vi "WaveGenerator_Sample_Program.vi"(0 "System no.":i32=1 min=1 step=1, 1 "Stop refnum":refnum<vi>, 2 "Affected axis":string="1", 3 "Selection":T1, 4 "DDL":bool, 5 "error in":errorcluster, 6 "Sine Parameters:":T3={"Xo (Start)"=0, "SIN_P Parameters"={"C"=200.0, "A"=10.0, "O"=0.0}, "N (Length)"=500, "Append? (&)"=FALSE} {"N (Length)" min=0 max=1000 step=1; "SIN_P Parameters"."O" format="%.6f"; "SIN_P Parameters"."A" format="%.6f"; "SIN_P Parameters"."C" format="%.6f"}, 7 "Ramp Parameters:":T2={"Xo (Start)"=0, "RAMP Parameters"={"C"=200.0, "J"=0.0, "A"=8.0, "O"=0.0}, "N (Length)"=500, "Append? (&)"=FALSE} {"N (Length)" min=0 max=1000 step=1; "RAMP Parameters"."O" format="%.6f"; "RAMP Parameters"."A" format="%.6f"; "RAMP Parameters"."J" format="%.6f"; "RAMP Parameters"."C" format="%.6f"}, 8 "Start position":dbl format="%.6f") -> (14 "Waveform":dbl[][](graph) caption="Graph showing the commanded (green) and measured (white) waveform and the position error (red).", 19 "Error out":errorcluster)   [LabVIEW 2014]
doc: "This VI demonstrates how to use the wave generator command VIs. It first moves the affected axis to a given start position. Then it runs in a loop, giving the user the options to write sine wave curve segments or ramps into the controllers wave buffer. Wave storage data points are limited to 1000 points to keep transfer times low. The segment length of one waveform - which normally defines the frequency - is predefined as 500 points in this example. Depending on the value of Append? (&), either the old buffer data is overwritten or the new wave will be appended to memory. Please take into account that you can append at most two waveforms since buffer size is limited to 1000 points as mentioned above. \n\nAdjust the following controls to modify the shape of the waveforms.\nN (Length): Waveform (i.e. the points to be modified) goes from 1 to Length. Datapoints from Length to 500 are filled with value of last wave point.\nXo (Start): Position where the first point of the waveform is located. \nC: Center point of the wave. If C = Length/2 then the wave is symmetrical.\nA: Amplitude of the waveform. F(x) = A*sin(x) + O\nO: Offset of the waveform. F(x) = A*sin(x) + O\nJ: Jerk. Means curvature in the transition to or from standstill.\n\nYou have to stop generator output prior to restarting it with a different parameter set. The Start Gen. and Stop Gen. buttons will enable or disable the wave generator output by sending \"WGO 0\" or \"WGO 1\" for the affected axis. If DDL is enabled \"WGO 65\" will be sent respectively. The red Stop button stops the wave generator output on the specified axis and finishes the loop. Please respect the delays that occur while the controller is processing your commands. This is indicated by the \"Busy?\" indicator. See manual for further details. \n\nIn case of an error a button Clear Error will appear and the control buttons above will be disabled. Pressing this button will clear the error status and enable the control buttons again.\nWith DDL ON you can achieve significantly better position accuracy. Compare the target (green), response (white) and error (red) signals on the graph. Since this is a very sensitive mechanism we recommend starting with low amplitudes and adjusting the parameters with caution. The DDL button works only if the controller supports DDL. Contact PI for information on activation of DDL support.\n\nSee User Manual for details about the use of the wave generator.\n\nRun XXXX_Configuration_Setup (with XXXX being the product number of your PI controller) prior to running this VI.\n\nValid for: E-712, E-725, E-727, E-753, E-754"
panel:
  out "Gen. running?":bool
  out "DDL":bool
  in  "Clear Error":bool
  out "Busy?":bool
  out "Controller error":bool
  in  "Stop":bool
  # "Wave generator sample program"
  # "This VI demonstrates how to use the wave generator command VIs. It first moves the affected axis to a given start position. Then it runs in a loop, giving the\nuser the options to write sine wave curve segments or ramps into the controllers wave buffer. Wave storage data points are limited to 1000 points\nto keep transfer times low. The segment length of one waveform is predefined as 500 points in this example. Depending on the value of Append? (&), either\nthe old buffer data is overwritten or the new wave will be appended to memory. You have to stop generator output prior to restarting it with a different\nparameter set. The Start Gen. and Stop Gen. buttons will enable or disable the wave generator output by sending \"WGO 0\" or \"WGO 1\" for the affected axis. \nIf DDL is enabled \"WGO 65\" will be sent respectively. The red Stop button stops the wave generator output on the specified axis and finishes the loop. Please\nrespect the delays that occur while the controller is processing your commands. This is indicated by the \"Busy?\" indicator. See manual for further details. \nRun XXXX_Configuration_Setup (with XXXX being the product number of your PI controller) prior to running this VI."
  # "DDL state"
  # "Stop VI\nand wave\ngenerator\noutput"
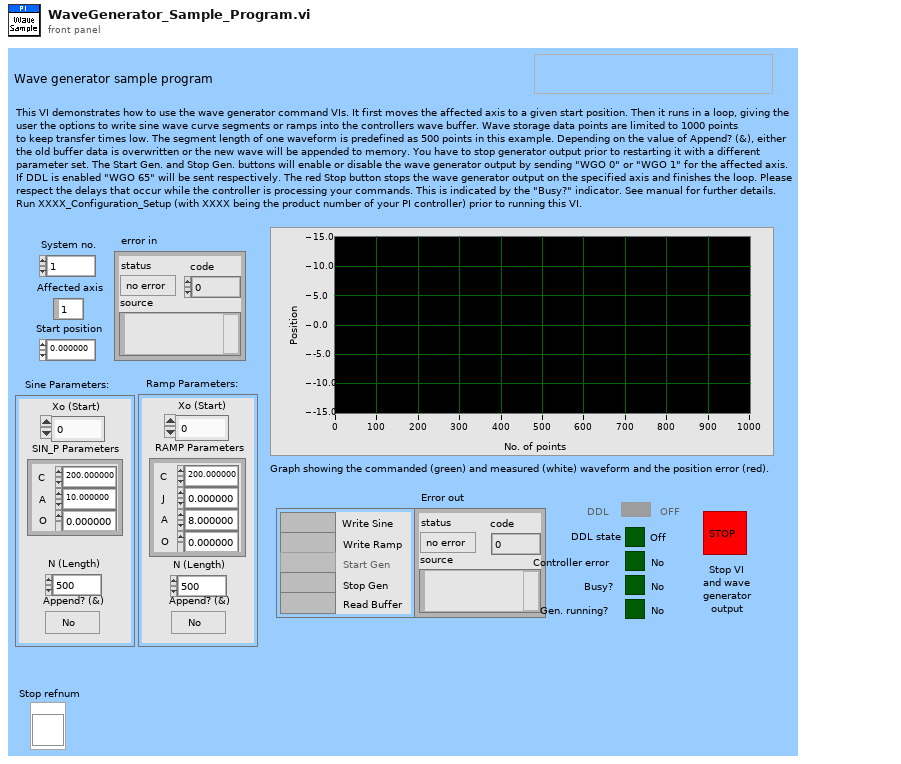
[diagram p1: front panel]
types:
  T1 = cluster{"Write Sine":bool, "Write Ramp":bool, "Start Gen":bool, "Stop Gen":bool, "Read Buffer":bool}
  T2 = cluster{"Xo (Start)":i32, "RAMP Parameters":cluster{"C":dbl, "J":dbl, "A":dbl, "O":dbl}, "N (Length)":i32, "Append? (&)":bool}
  T3 = cluster{"Xo (Start)":i32, "SIN_P Parameters":cluster{"C":dbl, "A":dbl, "O":dbl}, "N (Length)":i32, "Append? (&)":bool}
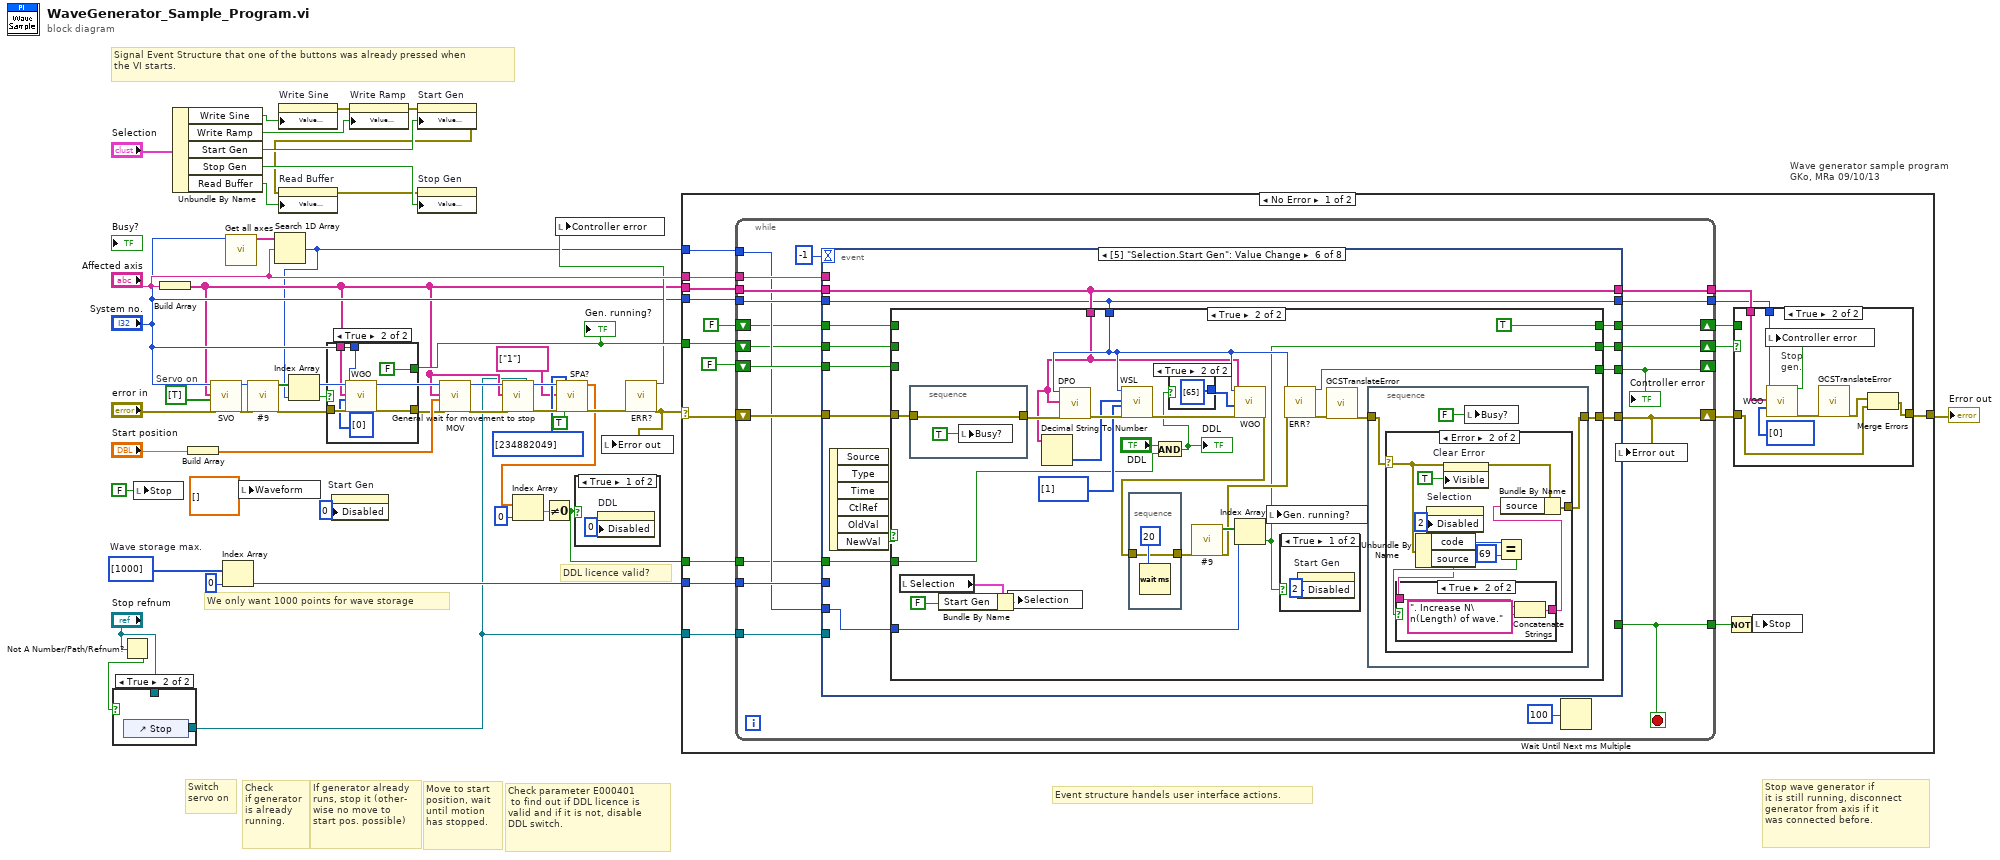
[diagram p0: block diagram]
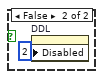
[diagram p2: hidden frame]
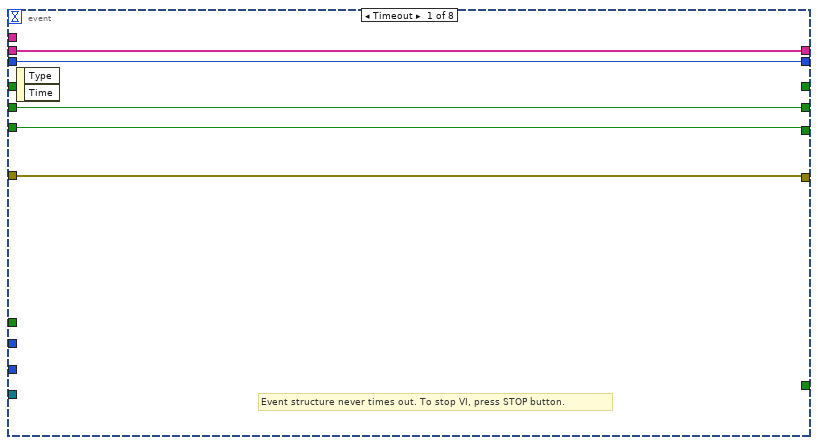
[diagram p6: hidden frame]
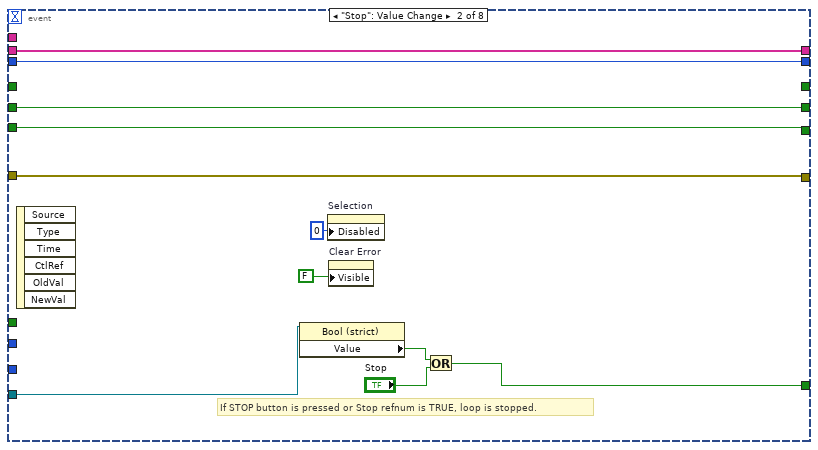
[diagram p7: hidden frame]
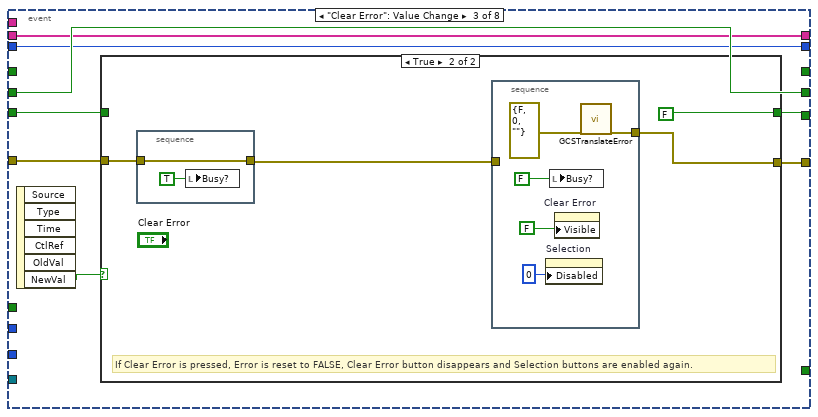
[diagram p8: hidden frame]
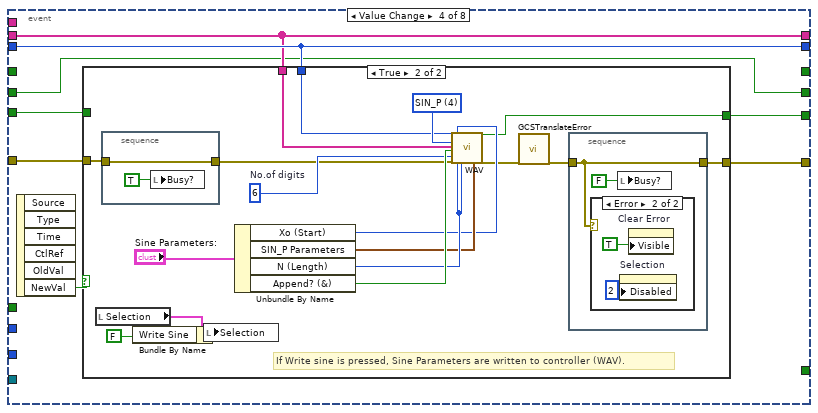
[diagram p10: hidden frame]
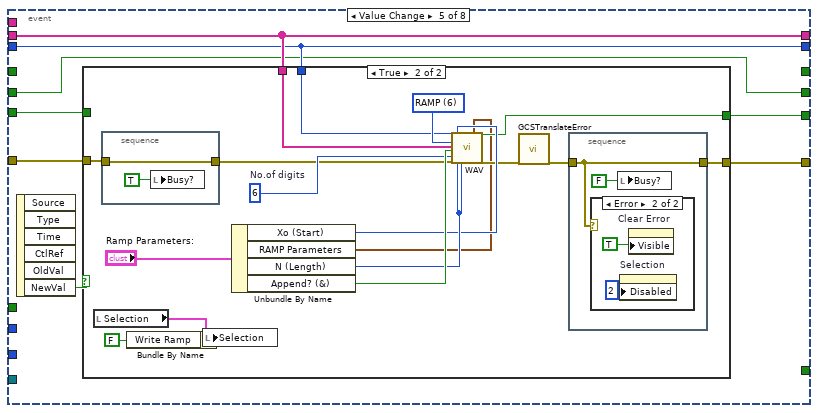
[diagram p13: hidden frame]
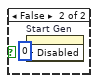
[diagram p17: hidden frame]
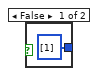
[diagram p18: hidden frame]
diagram:
  w44 = i32[] [1000]  # Wave storage max.
  # "Stop wave generator if\nit is still running, disconnect \ngenerator from axis if it\nwas connected before."
  # "Event structure handels user interface actions."
  # "Check parameter E000401\n to find out if DDL licence is\nvalid and if it is not, disable\nDDL switch."
  # "If generator already\nruns, stop it (other-\nwise no move to\nstart pos. possible)"
  # "Check\nif generator\nis already \nrunning."
  # "We only want 1000 points for wave storage"
  # "Switch\nservo on"
  # "Signal Event Structure that one of the buttons was already pressed when\nthe VI starts."
  # "DDL licence valid?"
  # "Servo on"
  # "Move to start\nposition, wait\nuntil motion\nhas stopped."
  # "Wave generator sample program\nGKo, MRa 09/10/13"
  n1 = Not A Number/Path/Refnum?(number/path/refnum="Stop refnum") -> (NaN/Path/Refnum?=w40:bool)
  n2 = case shown="True" w40 {
    tunnel: [w48 w49] -> w6
    tunnel: "Stop refnum" -> [w48 _]
    frame False {
    }
    frame True {
      n3 = control-ref of="Stop"() -> (w49:refnum<vi>)
    }
  }
  n4 = local write "Stop"(FALSE ("Controller error")) -> ()
  n5 = Build Array("Affected axis") -> (w20:string[])
  n6 = Unbundle By Name("Selection") -> ("Write Sine"=w11:bool, "Write Ramp"=w10:bool, "Start Gen"=w9:bool, "Stop Gen"=w8:bool, "Read Buffer"=w7:bool)
  n7 = Build Array("Start position") -> (w41:dbl[])
  n8 = call "SVO.vi"("System no."="System no.", "Axes to command"=w20, "Servo mode"=bool[] [TRUE], "error in"="error in") -> ("error out"=w34:errorcluster)  [unwired: 1 in, 14 out]
  n9 = Index Array(array=w44, index=0 ("Index")) -> (element=w45:i32)
  n10 = call "Get all axes.vi"("System no."="System no.") -> ("Conn. Axes"=w36:string[])  [unwired: 18 out]
  n11 = local write "Waveform"(dbl[][] [] ("Waveform")) -> ()
  n12 = call "#9.vi"("System no."="System no.", "error in"=w34) -> ("WG running?"=w37:bool[], "error out"=w29:errorcluster)  [unwired: 16 out]
  n13 = Search 1D Array(1D array=w36, element="Affected axis") -> (index of element=w16:i32)  [unwired: 1 out]
  n14 = property on="Write Sine" class="Bool (strict)"("Value (Signaling)"=w11) -> (error out=w5:errorcluster)  [unwired: 2 in, 1 out]
  n15 = Index Array(array=w37, index=w16) -> (element=w30:bool)
  n16 = case shown="True" w30 {
    selector: w30 -> [w51 _]
    tunnel: w29 -> [w50 w57]
    tunnel: [w50 w56] -> w28
    tunnel: "System no." -> [_ w54]
    tunnel: w20 -> [_ w53]
    tunnel: [w51 FALSE] -> w27
    frame False {
    }
    frame True {
      n17 = call "WGO.vi"("System no."=w54, "Affected axes"=w53, "WGO Parameter"=i32[] [0], "error in"=w57) -> ("error out"=w56:errorcluster)  [unwired: 15 out]
    }
  }
  "Gen. running?" <- w27
  n18 = property on="Start Gen" class="Bool (strict)"("Disabled"=u8 0) -> ()  [unwired: 2 in, 2 out]
  n19 = property on="Write Ramp" class="Bool (strict)"(error in=w5, "Value (Signaling)"=w10) -> (error out=w4:errorcluster)  [unwired: 1 in, 1 out]
  n20 = property on="Start Gen" class="Bool (strict)"(error in=w4, "Value (Signaling)"=w9) -> (error out=w3:errorcluster)  [unwired: 1 in, 1 out]
  n21 = property on="Stop Gen" class="Bool (strict)"(error in=w3, "Value (Signaling)"=w8) -> (error out=w2:errorcluster)  [unwired: 1 in, 1 out]
  n22 = property on="Read Buffer" class="Bool (strict)"(error in=w2, "Value (Signaling)"=w7) -> ()  [unwired: 1 in, 2 out]
  n23 = call "MOV.vi"("System no."="System no.", "Axes to move"=w20, "Position values"=w41, "error in"=w28) -> ("error out"=w31:errorcluster)  [unwired: 1 in, 14 out]
  n24 = call "General wait for movement to stop.vi"("System no."="System no.", "Axes to wait for"=w20, "error in"=w31, "Stop refnum"=w6) -> ("error out"=w22:errorcluster)  [unwired: 4 in, 11 out]
  n25 = call "SPA?.vi"("System no."="System no.", "Axes to query"=string[] ["1"], "error in"=w22, "Parameter no. (hex)"=u32[] [234882049], "Parameter no. format \n(Decimal: FALSE)"=TRUE ("Parameter no. format \n(Decimal: FALSE)")) -> ("Parameter value"=w17:dbl[], "error out"=w23:errorcluster)  [unwired: 2 in, 11 out]
  n26 = Index Array(array=w17, index=0) -> (element=w14:dbl)
  n27 = Not Equal To 0?(x=w14) -> (x != 0?=w13:bool)
  n28 = case shown="True" w13 {
    frame True {
      n29 = property on="DDL" class="Bool (strict)"("Disabled"=u8 0) -> ()  [unwired: 2 in, 2 out]
    }
    frame False {
      n30 = property on="DDL" class="Bool (strict)"("Disabled"=u8 2) -> ()  [unwired: 2 in, 2 out]
    }
  }
  n31 = call "ERR?.vi"("error in"=w23) -> ("Controller error"=w25:bool, "error out"=w26:errorcluster)  [unwired: 1 in, 16 out]
  n32 = local write "Controller error"(w25) -> ()
  n33 = local write "Error out"(w26) -> ()
  n34 = case shown="No Error" w26 {
    selector: w26 -> [w70 w376]
    tunnel: w20 -> [w78 _]
    tunnel: "System no." -> [w77 _]
    tunnel: [w68 w375] -> w47
    tunnel: w45 -> [w71 _]
    tunnel: "Affected axis" -> [w73 _]
    tunnel: w16 -> [w69 _]
    tunnel: w27 -> [w67 _]
    tunnel: w13 -> [w61 _]
    tunnel: w6 -> [w60 _]
    frame No Error {
      n35 = while {
        tunnel: w73 -> [w99]
        tunnel: w71 -> [w100]
        shift-left: w70 -> [w102]
        shift-right: [w101] -> w74
        tunnel: [w103] -> w75
        tunnel: [w105] -> w76
        tunnel: w77 -> [w104]
        tunnel: w78 -> [w106]
        shift-right: [w97] -> _
        shift-left: FALSE ("Controller error") -> [w96]
        tunnel: w69 -> [w95]
        shift-right: [w93] -> w66
        shift-left: w67 -> [w94]
        tunnel: [w92] -> w65
        shift-right: [w91] -> w62
        shift-left: FALSE -> [w90]
        tunnel: w61 -> [w89]
        tunnel: w60 -> [w88]
        stop <- w92 stop-if-true
        n36 = event shown="[5] \"Selection.Start Gen\": Value Change" {
          selector: _ -> [_ _ _ _ _ _ _ _]
          dyn-events: _ -> [_ _ _ _ _ _ _ _]
          timeout: -1 -> [_ _ _ _ _ _ _ _]
          tunnel: w106 -> [w110 w121 w124 w146 w181 w220 w284 w323]
          tunnel: [w110 w121 w124 w146 w181 w220 w284 w323] -> w105
          tunnel: w104 -> [w109 w120 w125 w147 w180 w219 w283 w324]
          tunnel: [w109 w120 w125 w147 w180 w219 w283 w324] -> w103
          tunnel: w102 -> [w111 w122 w127 w150 w184 w223 w288 w330]
          tunnel: [w111 w122 w128 w151 w185 w224 w289 w331] -> w101
          tunnel: w100 -> [_ _ _ _ _ _ _ w325]
          tunnel: w99 -> [_ _ _ _ _ _ _ w326]
          tunnel: [w112 w123 w129 w152 w186 w225 w290 w332] -> w97
          tunnel: w96 -> [w112 w123 w130 w148 w182 w221 w286 w328]
          tunnel: w95 -> [_ _ _ _ _ w213 w285 w327]
          tunnel: [_ w115 _ _ _ _ _ _] -> w92
          tunnel: w94 -> [w108 w119 w126 w145 w179 w217 w281 w322]
          tunnel: [w108 w119 w126 w145 w179 w218 w282 w322] -> w93
          tunnel: [_ _ _ _ _ w216 _ _] -> w91
          tunnel: w90 -> [_ _ _ _ _ w215 _ _]
          tunnel: w89 -> [_ _ _ _ _ w214 _ _]
          tunnel: w88 -> [_ w118 _ _ _ _ _ _]
          event Timeout {
            # "Event structure never times out. To stop VI, press STOP button."
            n37 = event-data() -> ()  [unwired: 3 out]
          }
          event "Stop": Value Change {
            # "If STOP button is pressed or Stop refnum is TRUE, loop is stopped."
            n38 = event-data() -> ()  [unwired: 7 out]
            n39 = property class="Bool (strict)"(reference=w118) -> ("Value"=w117:bool)  [unwired: 1 in, 2 out]
            n40 = property on="Selection" class="Clust (strict)"("Disabled"=u8 0) -> ()  [unwired: 2 in, 2 out]
            n41 = property on="Clear Error" class="Bool"("Visible"=FALSE) -> ()  [unwired: 2 in, 2 out]
            n42 = Or(x=w117, y="Stop") -> (x .or. y?=w115:bool)
          }
          event "Clear Error": Value Change {
            n43 = event-data() -> ("NewVal"=w131:bool)  [unwired: 6 out]
            n44 = case shown="True" w131 {
              tunnel: w130 -> [w133 _]
              tunnel: [w133 FALSE ("Controller error")] -> w129
              tunnel: [w132 w135] -> w128
              tunnel: w127 -> [w132 w136]
              frame False {
              }
              frame True {
                # "If Clear Error is pressed, Error is reset to FALSE, Clear Error button disappears and Selection buttons are enabled again."
                n45 = stacked-sequence {
                  tunnel: w136 -> [w143]
                  tunnel: [w143] -> w134
                  frame #0 {
                    n46 = local write "Busy?"(TRUE) -> ()
                  }
                }
                n47 = stacked-sequence {
                  tunnel: [w138] -> w135
                  tunnel: w134 -> [_]
                  frame #0 {
                    n48 = property on="Selection" class="Clust (strict)"("Disabled"=u8 0) -> ()  [unwired: 2 in, 2 out]
                    n49 = local write "Busy?"(FALSE) -> ()
                    n50 = property on="Clear Error" class="Bool"("Visible"=FALSE) -> ()  [unwired: 2 in, 2 out]
                    n51 = call "GCSTranslateError.vi"("error in"=errorcluster {"status"=FALSE, "code"=0, "source"=""} ("error IO")) -> ("error out"=w138:errorcluster)  [unwired: 18 out]
                  }
                }
              }
            }
          }
          event "Selection.Write Sine": Value Change {
            n52 = event-data() -> ("NewVal"=w149:bool)  [unwired: 6 out]
            n53 = case shown="True" w149 {
              tunnel: [w153 w165] -> w152
              tunnel: w147 -> [_ w157]
              tunnel: w146 -> [_ w156]
              tunnel: [w154 w162] -> w151
              tunnel: w150 -> [w154 w161]
              tunnel: w148 -> [w153 _]
              frame False {
              }
              frame True {
                w168 = i16 6  # No.of digits
                w167 = u16 4 items=["SIN", "POL", "TAN", "PNT", "SIN_P", "LIN", "RAMP"] ("Waveform")
                # "If Write sine is pressed, Sine Parameters are written to controller (WAV)."
                n54 = local read "Selection"() -> (w160:T1)
                n55 = stacked-sequence {
                  tunnel: w161 -> [w173]
                  tunnel: [w173] -> w155
                  frame #0 {
                    n56 = local write "Busy?"(TRUE) -> ()
                  }
                }
                n57 = Bundle By Name(cluster=w160, "Write Sine"=FALSE) -> (w159:T1)
                n58 = local write "Selection"(w159) -> ()
                n59 = Unbundle By Name("Sine Parameters:") -> ("Xo (Start)"=w169:i32, "SIN_P Parameters"=w170:cluster{"C":dbl, "A":dbl, "O":dbl}, "N (Length)"=w171:i32, "Append? (&)"=w172:bool)
                n60 = call "WAV.vi"("System no."=w157, "Waveform"=w167, "Affected axes"=w156, "Append? (&)"=w172, "No.of digits"=w168, "error in"=w155, "Xo"=w169, "N"=w171, "Segment length"=w171, "SIN_P Parameters"=w170) -> ("Controller error"=w165:bool, "error out"=w164:errorcluster)  [unwired: 10 in, 6 out]
                n61 = call "GCSTranslateError.vi"("error in"=w164) -> ("error out"=w163:errorcluster)  [unwired: 18 out]
                n62 = stacked-sequence {
                  tunnel: w163 -> [w175]
                  tunnel: [w175] -> w162
                  frame #0 {
                    n63 = case shown="Error" w175 {
                      frame No Error {
                      }
                      frame Error {
                        n64 = property on="Selection" class="Clust (strict)"("Disabled"=u8 2) -> ()  [unwired: 2 in, 2 out]
                        n65 = property on="Clear Error" class="Bool"("Visible"=TRUE) -> ()  [unwired: 2 in, 2 out]
                      }
                    }
                    n66 = local write "Busy?"(FALSE) -> ()
                  }
                }
              }
            }
          }
          event "Selection.Write Ramp": Value Change {
            n67 = event-data() -> ("NewVal"=w183:bool)  [unwired: 6 out]
            n68 = case shown="True" w183 {
              tunnel: [w187 w201] -> w186
              tunnel: w180 -> [_ w200]
              tunnel: w181 -> [_ w199]
              tunnel: [w188 w196] -> w185
              tunnel: w184 -> [w188 w195]
              tunnel: w182 -> [w187 _]
              frame False {
              }
              frame True {
                w203 = i16 6  # No.of digits
                w202 = u16 6 items=["SIN", "POL", "TAN", "PNT", "SIN_P", "LIN", "RAMP"] ("Waveform")
                n69 = local read "Selection"() -> (w191:T1)
                n70 = stacked-sequence {
                  tunnel: w195 -> [w207]
                  tunnel: [w207] -> w194
                  frame #0 {
                    n71 = local write "Busy?"(TRUE) -> ()
                  }
                }
                n72 = Bundle By Name(cluster=w191, "Write Ramp"=FALSE ("Write Sine")) -> (w190:T1)
                n73 = local write "Selection"(w190) -> ()
                n74 = Unbundle By Name("Ramp Parameters:") -> ("Xo (Start)"=w204:i32, "RAMP Parameters"=w192:cluster{"C":dbl, "J":dbl, "A":dbl, "O":dbl}, "N (Length)"=w205:i32, "Append? (&)"=w206:bool)
                n75 = call "WAV.vi"("System no."=w200, "Waveform"=w202, "Affected axes"=w199, "Append? (&)"=w206, "No.of digits"=w203, "error in"=w194, "Xo"=w204, "N"=w205, "Segment length"=w205, "RAMP Parameters"=w192) -> ("Controller error"=w201:bool, "error out"=w198:errorcluster)  [unwired: 10 in, 6 out]
                n76 = call "GCSTranslateError.vi"("error in"=w198) -> ("error out"=w197:errorcluster)  [unwired: 18 out]
                n77 = stacked-sequence {
                  tunnel: w197 -> [w209]
                  tunnel: [w209] -> w196
                  frame #0 {
                    n78 = case shown="Error" w209 {
                      frame No Error {
                      }
                      frame Error {
                        n79 = property on="Selection" class="Clust (strict)"("Disabled"=u8 2) -> ()  [unwired: 2 in, 2 out]
                        n80 = property on="Clear Error" class="Bool"("Visible"=TRUE) -> ()  [unwired: 2 in, 2 out]
                      }
                    }
                    n81 = local write "Busy?"(FALSE) -> ()
                  }
                }
              }
            }
          }
          event "Selection.Start Gen": Value Change {
            n82 = event-data() -> ("NewVal"=w222:bool)  [unwired: 6 out]
            n83 = case shown="True" w222 {
              tunnel: [w228 w245] -> w225
              tunnel: w219 -> [_ w244]
              tunnel: w220 -> [_ w243]
              tunnel: [w229 w254] -> w224
              tunnel: w223 -> [w229 w253]
              tunnel: w221 -> [w228 _]
              tunnel: [w227 w238] -> w218
              tunnel: w217 -> [w227 _]
              tunnel: [w226 TRUE] -> w216
              tunnel: w215 -> [w226 _]
              tunnel: w214 -> [_ w232]
              tunnel: w213 -> [_ w230]
              frame False {
              }
              frame True {
                n84 = local read "Selection"() -> (w237:T1)
                n85 = stacked-sequence {
                  tunnel: w253 -> [w262]
                  tunnel: [w262] -> w247
                  frame #0 {
                    n86 = local write "Busy?"(TRUE) -> ()
                  }
                }
                n87 = Bundle By Name(cluster=w237, "Start Gen"=FALSE ("Write Sine")) -> (w236:T1)
                n88 = local write "Selection"(w236) -> ()
                n89 = Decimal String To Number(string=w243) -> (number=w248:i32[])  [unwired: 3 out]
                n90 = call "DPO.vi"("System no."=w244, "DPO axes"=w243, "error in"=w247) -> ("error out"=w250:errorcluster)  [unwired: 2 in, 14 out]
                n91 = call "WSL.vi"("System no."=w244, "Generator ID"=w248, "WaveTableID"=i32[] [1], "error in"=w250) -> ("error out"=w251:errorcluster)  [unwired: 15 out]
                n92 = And(x="DDL", y=w232) -> (x .and. y?=w231:bool)
                "DDL" <- w231
                n93 = case shown="True" w231 {
                  tunnel: [i32[] [1] ("WGO Parameter") i32[] [65] ("WGO Parameter")] -> w252
                  frame False {
                  }
                  frame True {
                  }
                }
                n94 = call "WGO.vi"("System no."=w244, "Affected axes"=w243, "WGO Parameter"=w252, "error in"=w251) -> ("error out"=w240:errorcluster)  [unwired: 15 out]
                n95 = stacked-sequence {
                  tunnel: w240 -> [w258]
                  tunnel: [w258] -> w242
                  frame #0 {
                    n96 = Wait (ms)(milliseconds to wait=u32 20) -> ()  [unwired: 1 out]
                  }
                }
                n97 = call "#9.vi"("error in"=w242) -> ("WG running?"=w241:bool[], "error out"=w239:errorcluster)  [unwired: 1 in, 16 out]
                n98 = Index Array(array=w241, index=w230) -> (element=w238:bool)
                n99 = local write "Gen. running?"(w238) -> ()
                n100 = case shown="True" w238 {
                  frame True {
                    n101 = property on="Start Gen" class="Bool (strict)"("Disabled"=u8 2) -> ()  [unwired: 2 in, 2 out]
                  }
                  frame False {
                    n102 = property on="Start Gen" class="Bool (strict)"("Disabled"=u8 0) -> ()  [unwired: 2 in, 2 out]
                  }
                }
                n103 = call "ERR?.vi"("System no."=w244, "error in"=w239) -> ("Controller error"=w245:bool, "error out"=w246:errorcluster)  [unwired: 16 out]
                n104 = call "GCSTranslateError.vi"("error in"=w246) -> ("error out"=w255:errorcluster)  [unwired: 18 out]
                n105 = stacked-sequence {
                  tunnel: w255 -> [w265]
                  tunnel: [w264] -> w254
                  frame #0 {
                    n106 = case shown="Error" w265 {
                      selector: w265 -> [w267 w272]
                      tunnel: [w267 w270] -> w264
                      frame No Error {
                      }
                      frame Error {
                        n107 = Unbundle By Name(w272) -> ("code"=w274:i32, "source"=w268:string)
                        n108 = property on="Selection" class="Clust (strict)"("Disabled"=u8 2) -> ()  [unwired: 2 in, 2 out]
                        n109 = property on="Clear Error" class="Bool"("Visible"=TRUE) -> ()  [unwired: 2 in, 2 out]
                        n110 = Equal?(x=w274, y=69) -> (x = y?=w269:bool)
                        n111 = case shown="True" w269 {
                          tunnel: [w277 w279] -> w271
                          tunnel: w268 -> [w277 w278]
                          frame False {
                          }
                          frame True {
                            n112 = Concatenate Strings(w278, ". Increase N\n(Length) of wave.") -> (w279:string)
                          }
                        }
                        n113 = Bundle By Name(cluster=w272, "source"=w271) -> (w270:errorcluster)
                      }
                    }
                    n114 = local write "Busy?"(FALSE) -> ()
                  }
                }
              }
            }
          }
          event "Selection.Stop Gen": Value Change {
            n115 = event-data() -> ("NewVal"=w287:bool)  [unwired: 6 out]
            n116 = case shown="True" w287 {
              tunnel: [w292 w306] -> w290
              tunnel: w283 -> [_ w300]
              tunnel: w284 -> [_ w305]
              tunnel: [w293 w310] -> w289
              tunnel: w288 -> [w293 w309]
              tunnel: w286 -> [w292 _]
              tunnel: w285 -> [_ w298]
              tunnel: [w291 w297] -> w282
              tunnel: w281 -> [w291 _]
              frame False {
              }
              frame True {
                n117 = local read "Selection"() -> (w296:T1)
                n118 = stacked-sequence {
                  tunnel: w309 -> [w316]
                  tunnel: [w316] -> w304
                  frame #0 {
                    n119 = local write "Busy?"(TRUE) -> ()
                  }
                }
                n120 = Bundle By Name(cluster=w296, "Stop Gen"=FALSE ("Write Sine")) -> (w295:T1)
                n121 = local write "Selection"(w295) -> ()
                n122 = call "WGO.vi"("System no."=w300, "Affected axes"=w305, "WGO Parameter"=i32[] [0], "error in"=w304) -> ("error out"=w303:errorcluster)  [unwired: 15 out]
                n123 = stacked-sequence {
                  tunnel: w303 -> [w314]
                  tunnel: [w314] -> w302
                  frame #0 {
                    n124 = Wait (ms)(milliseconds to wait=u32 20) -> ()  [unwired: 1 out]
                  }
                }
                n125 = call "#9.vi"("System no."=w300, "error in"=w302) -> ("WG running?"=w299:bool[], "error out"=w301:errorcluster)  [unwired: 16 out]
                n126 = Index Array(array=w299, index=w298) -> (element=w297:bool)
                n127 = local write "Gen. running?"(w297) -> ()
                n128 = case shown="True" w297 {
                  frame True {
                    n129 = property on="Start Gen" class="Bool (strict)"("Disabled"=u8 2) -> ()  [unwired: 2 in, 2 out]
                  }
                  frame False {
                    n130 = property on="Start Gen" class="Bool (strict)"("Disabled"=u8 0) -> ()  [unwired: 2 in, 2 out]
                  }
                }
                n131 = call "ERR?.vi"("System no."=w300, "error in"=w301) -> ("Controller error"=w306:bool, "error out"=w307:errorcluster)  [unwired: 16 out]
                n132 = call "GCSTranslateError.vi"("error in"=w307) -> ("error out"=w311:errorcluster)  [unwired: 18 out]
                n133 = stacked-sequence {
                  tunnel: w311 -> [w318]
                  tunnel: [w318] -> w310
                  frame #0 {
                    n134 = case shown="Error" w318 {
                      frame No Error {
                      }
                      frame Error {
                        n135 = property on="Selection" class="Clust (strict)"("Disabled"=u8 2) -> ()  [unwired: 2 in, 2 out]
                        n136 = property on="Clear Error" class="Bool"("Visible"=TRUE) -> ()  [unwired: 2 in, 2 out]
                      }
                    }
                    n137 = local write "Busy?"(FALSE) -> ()
                  }
                }
              }
            }
          }
          event "Selection.Read Buffer": Value Change {
            n138 = event-data() -> ("NewVal"=w329:bool)  [unwired: 6 out]
            n139 = case shown="True" w329 {
              tunnel: [w333 w344] -> w332
              tunnel: w324 -> [_ w341]
              tunnel: w323 -> [_ _]
              tunnel: [w334 w367] -> w331
              tunnel: w330 -> [w334 w366]
              tunnel: w328 -> [w333 _]
              tunnel: w327 -> [_ _]
              tunnel: w326 -> [_ w340]
              tunnel: w325 -> [_ w338]
              frame False {
              }
              frame True {
                w352 = 3 ("Numeric")
                w353 = 2 ("Numeric")
                w360 = 1 ("Numeric")
                # "Record and display values"
                n140 = stacked-sequence {
                  tunnel: w366 -> [w369]
                  tunnel: [w369] -> w342
                  frame #0 {
                    n141 = local write "Busy?"(TRUE) -> ()
                  }
                }
                n142 = call "DRC.vi"("System no."=w341, "Rec. table"=w360, "Rec. option"=w360, "error in"=w342, "Source ID"=w340) -> ("Controller error"=w350:bool, "error out"=w359:errorcluster)  [unwired: 1 in, 12 out]
                n143 = call "DRC.vi"("System no."=w341, "Rec. table"=w353, "Rec. option"=w353, "error in"=w359, "Source ID"=w340) -> ("Controller error"=w349:bool, "error out"=w358:errorcluster)  [unwired: 1 in, 12 out]
                n144 = call "DRC.vi"("System no."=w341, "Rec. table"=w352, "Rec. option"=w352, "error in"=w358, "Source ID"=w340) -> ("Controller error"=w348:bool, "error out"=w351:errorcluster)  [unwired: 1 in, 12 out]
                n145 = call "WGR.vi"("System no."=w341, "error in"=w351) -> ("error out"=w346:errorcluster)  [unwired: 2 in, 15 out]
                n146 = call "DRR?.vi"("System no."=w341, "Rec. table IDs"=i32[] [1, 2, 3], "error in"=w346, "Xo"=1, "N"=w338, "Nmax"=w338) -> ("Data"=w363:dbl[][], "error out"=w343:errorcluster)  [unwired: 2 in, 10 out]
                n147 = Index Array(array=w363, index (col) #1=0 ("Disabled Index (col)"), index (col) #2=1 ("Disabled Index (col)"), index (col) #3=2 ("Disabled Index (col)")) -> (element #1=w361:dbl[], element #2=w355:dbl[], element #3=w354:dbl[])  [unwired: 3 in]
                n148 = Build Array(w361, w355, w354) -> (→"Waveform":dbl[][])
                n149 = call "ERR?.vi"("System no."=w341, "error in"=w343) -> ("Controller error"=w345:bool, "error out"=w365:errorcluster)  [unwired: 16 out]
                n150 = call "GCSTranslateError.vi"("error in"=w365) -> ("error out"=w368:errorcluster)  [unwired: 18 out]
                n151 = Compound Arithmetic op=OR(w345, w350, w349, w348) -> (w344:bool)
                n152 = local read "Selection"() -> (w337:T1)
                n153 = stacked-sequence {
                  tunnel: w368 -> [w371]
                  tunnel: [w371] -> w367
                  frame #0 {
                    n154 = case shown="Error" w371 {
                      frame No Error {
                      }
                      frame Error {
                        n155 = property on="Selection" class="Clust (strict)"("Disabled"=u8 2) -> ()  [unwired: 2 in, 2 out]
                        n156 = property on="Clear Error" class="Bool"("Visible"=TRUE) -> ()  [unwired: 2 in, 2 out]
                      }
                    }
                    n157 = local write "Busy?"(FALSE) -> ()
                  }
                }
                n158 = Bundle By Name(cluster=w337, "Read Buffer"=FALSE ("Write Sine")) -> (w336:T1)
                n159 = local write "Selection"(w336) -> ()
              }
            }
          }
        }
        "Controller error" <- w97
        n160 = Wait Until Next ms Multiple(millisecond multiple=u32 100) -> ()  [unwired: 1 out]
        n161 = local write "Error out"(w101) -> ()
      }
      n162 = Not(x=w65) -> (.not. x?=w64:bool)
      n163 = case shown="True" w66 {
        tunnel: w76 -> [_ w84]
        tunnel: w75 -> [_ w85]
        tunnel: w74 -> [w79 w81]
        tunnel: [w79 w83] -> w68
        tunnel: w62 -> [_ _]
        frame False {
        }
        frame True {
          # "Stop\ngen."
          n164 = call "WGO.vi"("System no."=w85, "Affected axes"=w84, "WGO Parameter"=i32[] [0] ("WGO \nParameter")) -> ("Controller error"=w86:bool, "error out"=w80:errorcluster)  [unwired: 1 in, 14 out]
          n165 = local write "Controller error"(w86) -> ()
          n166 = call "GCSTranslateError.vi"("error in"=w80) -> ("error out"=w82:errorcluster)  [unwired: 18 out]
          n167 = Merge Errors(w82, w81) -> (w83:errorcluster)
        }
      }
      n168 = local write "Stop"(w64) -> ()
    }
    frame Error {
      n169 = call "GCSTranslateError.vi"("error in"=w376) -> ("error out"=w375:errorcluster)  [unwired: 18 out]
    }
  }
  "Error out" <- w47
